vi "Ping.vi"(8 "error in (no error)":errorcluster, 11 "mqtt in":refnum<class "MQTT Client.lvclass">) -> (0 "error out":errorcluster, 3 "mqtt out":refnum<class "MQTT Client.lvclass">)   [LabVIEW 2020, in "MQTT Client.lvclass"]
uses:
  MQTT Client.lvclass
  mqttCmd/mqttCmdPing/PingMqttMsg.lvclass
  C:/Projects/Libraries/Gore SM 2020/mqtt-LabVIEW/src/class/mqtt/mqttCmd/BaseMqttMsg.lvclass
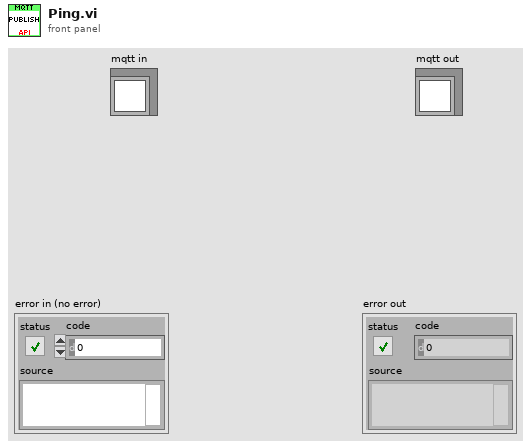
[diagram p1: front panel]
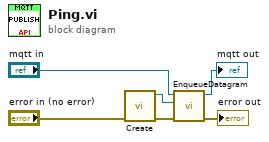
[diagram p0: block diagram]
diagram:
  n1 = call "Create.vi"("error in (no error)"="error in (no error)") -> ("error out"=w2:errorcluster, "mqttCmdPing out"=w3:refnum<class "PingMqttMsg.lvclass">)  [unwired: 9 in]
  n2 = call "EnqueueDatagram.vi"("error in (no error)"=w2, "mqttCmd"=w3, "mqtt in"="mqtt in") -> ("error out"=→"error out":errorcluster, "mqtt out"=→"mqtt out":refnum<class "MQTT Client.lvclass">)  [unwired: 7 in]
